vi "InitLinkedList.vi"(9 "Names":string[](array[string]), 11 "LinkedList in":T1) -> (3 "LinkedList out":T1)   [LabVIEW 2010]
uses:
  LinkedList.ctl
  Node.ctl
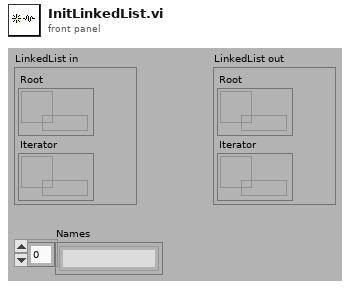
[diagram p1: front panel]
types:
  T1 = typedef "LinkedList.ctl" = cluster{"Root":refnum<data-value>, "Iterator":refnum<data-value>}
  T2 = typedef "Node.ctl" = cluster{"Name":string, "Next":variant, "Previous":variant}
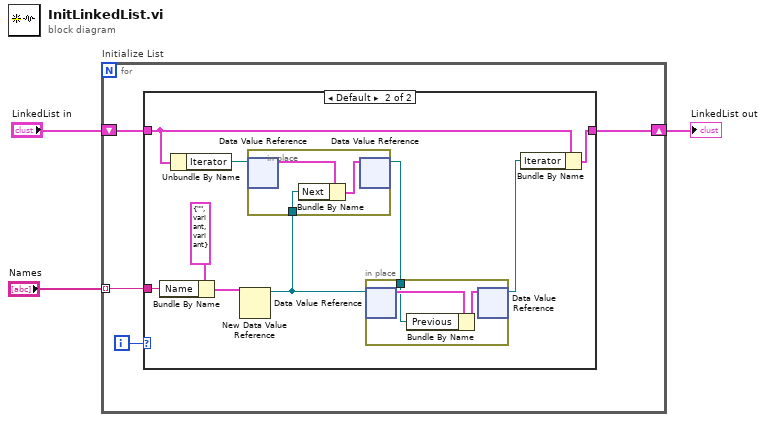
[diagram p0: block diagram]
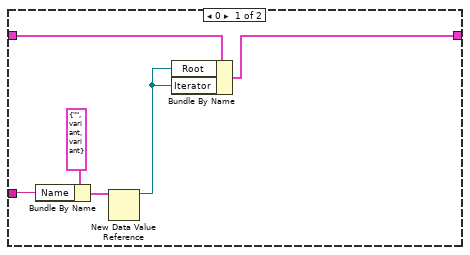
[diagram p2: hidden frame]
diagram:
  n1 = for "Initialize List" {
    shift-right: [w4] -> w3
    shift-left: "LinkedList in" -> [w6]
    tunnel: "Names" -> [w5] mode=indexing
    i -> [w7]
    n2 = case shown="Default" w7 {
      tunnel: w6 -> [w13 w16]
      tunnel: w5 -> [w11 w21]
      tunnel: [w10 w15] -> w4
      frame 0 {
        n3 = Bundle By Name(cluster=T2 {"Name"="", "Next"=variant, "Previous"=variant} ("Data"), "Name"=w11) -> (w9:T2)
        n4 = New Data Value Reference(data value=w9) -> (data value reference=w8:refnum<data-value>)  [unwired: 1 in, 1 out]
        n5 = Bundle By Name(cluster=w13, "Root"=w8, "Iterator"=w8) -> (w10:T1)
      }
      frame Default {
        n6 = Bundle By Name(cluster=T2 {"Name"="", "Next"=variant, "Previous"=variant} ("Data"), "Name"=w21) -> (w20:T2)
        n7 = Unbundle By Name(w16) -> ("Iterator"=w19:refnum<data-value>)
        n8 = New Data Value Reference(data value=w20) -> (data value reference=w18:refnum<data-value>)  [unwired: 1 in, 1 out]
        n9 = in-place {
          in-place-border: w18 -> [w27]
          n10 = in-place-dvr #1(w19) -> (w28:T2)  [unwired: 1 out]
          n11 = Bundle By Name(cluster=w28, "Next"=w27) -> (w26:T2)
          n12 = in-place-dvr #1(w26) -> (w17:refnum<data-value>)  [unwired: 1 out]
        }
        n13 = in-place {
          in-place-border: w17 -> [w23]
          n14 = in-place-dvr #2(w18) -> (w25:T2)  [unwired: 1 out]
          n15 = Bundle By Name(cluster=w25, "Previous"=w23) -> (w24:T2)
          n16 = in-place-dvr #2(w24) -> (w14:refnum<data-value>)  [unwired: 1 out]
        }
        n17 = Bundle By Name(cluster=w16, "Iterator"=w14) -> (w15:T1)
      }
    }
  }
  "LinkedList out" <- w3
